vi "pll-read.vi"(8 "error in (no error)":errorcluster, 11 "PLL reader.lvclass":refnum<class "PLL reader.lvclass">) -> (0 "error out":errorcluster, 2 "Result":dbl[](array[numeric]), 3 "PLL reader.lvclass Out":refnum<class "PLL reader.lvclass">)   [LabVIEW 2020, in "PLL reader.lvclass"]
uses:
  PLL reader.lvclass
  opt/github/NHMFL_Core/Libraries/Instruments/Instrument Driver/Instrument Driver.lvclass
  resonant_ultrasound_arxiv/maglab ultrasound -- arkady --arxiv/publisher action.ctl
  NHMFL_Core/Libraries/Instruments/Instrument Driver/Instrument Driver.lvclass/Instrument Driver.ctl
  NHMFL_Core/Libraries/Instruments/Instrument Driver/Write Channel names.vi
  NHMFL_Core/Libraries/Instruments/Instrument Driver/Write Channel units.vi
  PLL reader.lvclass/PLL reader.ctl
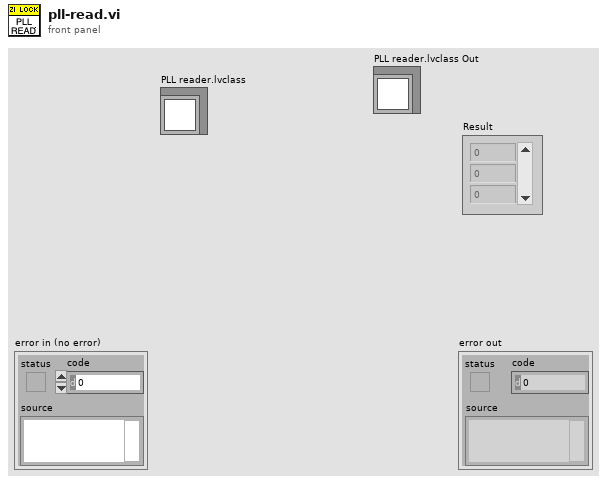
[diagram p1: front panel]
types:
  T1 = typedef "publisher action.ctl" = enum16{"set", "get", "init", "check"}
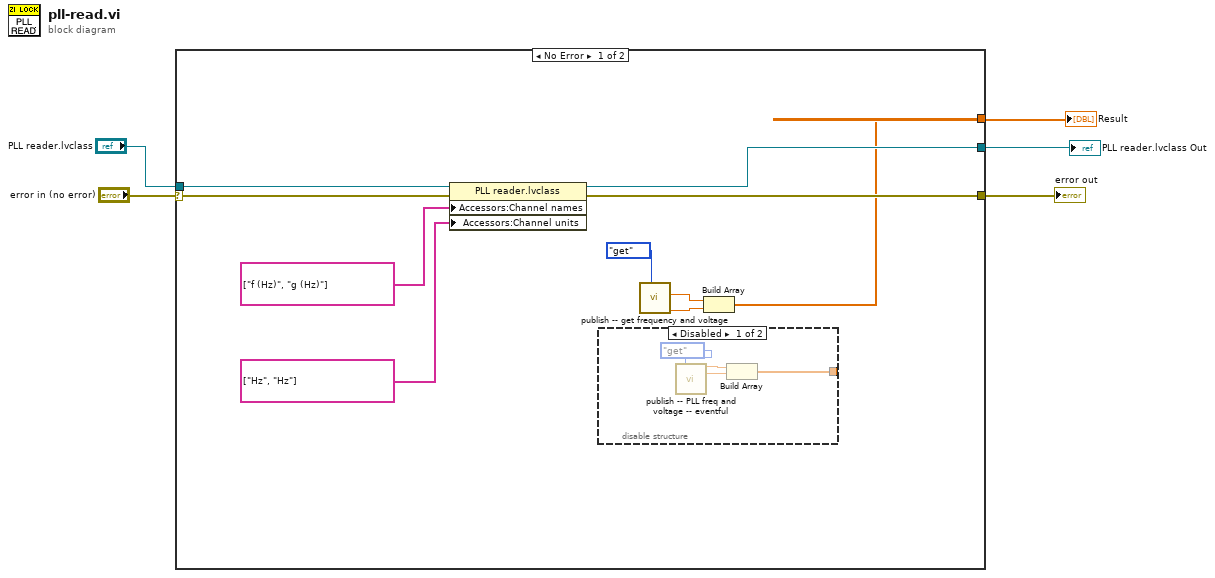
[diagram p0: block diagram]
diagram:
  n1 = case shown="No Error" "error in (no error)" {
    selector: "error in (no error)" -> [w13 w21]
    tunnel: [w12 w21] -> w4
    tunnel: [w14 w20] -> w2
    tunnel: "PLL reader.lvclass" -> [w15 w20]
    tunnel: [w6 _] -> w3
    frame No Error {
      n2 = property class="PLL reader.lvclass"(reference=w15, error in=w13, "Accessors:Channel names"=string[] ["f (Hz)", "g (Hz)"] ("Channel names"), "Accessors:Channel units"=string[] ["Hz", "Hz"] ("Channel names")) -> (reference out=w14:refnum<class "PLL reader.lvclass">, error out=w12:errorcluster)
      n3 = disable-structure shown="Disabled" {
        disable-tunnel: [w16 _] -> _
        frame Disabled {
          n4 = call "publish -- PLL freq and voltage -- eventful.vi"("publisher action"=publisher_action."get") -> ("freq out (Hz)"=w18:dbl, "gamma OUT (Hz)"=w17:dbl)  [unwired: 9 in, 4 out]
          n5 = Build Array(w18, w17) -> (w16:dbl[])
        }
        frame Enabled {
        }
      }
      n6 = call "publish -- get frequency and voltage.vi"("publisher action"=publisher_action."get") -> ("gamma OUT (Hz)"=w7:dbl, "freq out (Hz)"=w8:dbl)  [unwired: 8 in, 1 out]
      n7 = Build Array(w8, w7) -> (w6:dbl[])
    }
    frame Error {
    }
  }
  "error out" <- w4
  "Result" <- w3
  "PLL reader.lvclass Out" <- w2
